vi "WordOfTheDay.vi"() -> ()   [LabVIEW 2018]
uses:
  State.ctl
  <vilib>/Utility/error.llb/Error Cluster From Error Code.vi
  <vilib>/ErrorRing/Error Ring.xnode
  MerriamWebsterJSON.lvlib
panel:
  out "error out":errorcluster
  in  "error in (no error)":errorcluster
  out "Audio Found?":bool
  in  "Play Sound":bool
  in  "Get Word":bool
  out "Output":string
  in  "Stop":bool
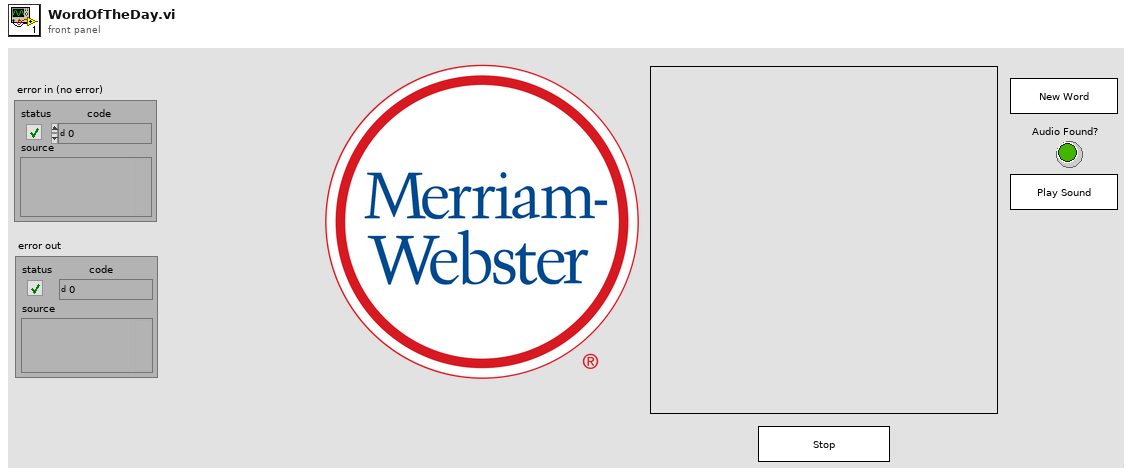
[diagram p1: front panel]
types:
  T1 = typedef "State.ctl" = enum16{"Init", "Wait", "Get Definition", "Get Sound", "Play Sound", "Shutdown"}
  T2 = enum8{"Enabled", "Disabled", "Disabled and Grayed Out"}
  T3 = typedef "LabVIEWHTTPClient.lvlib/ClientHandle.ctl" = refnum<k1>
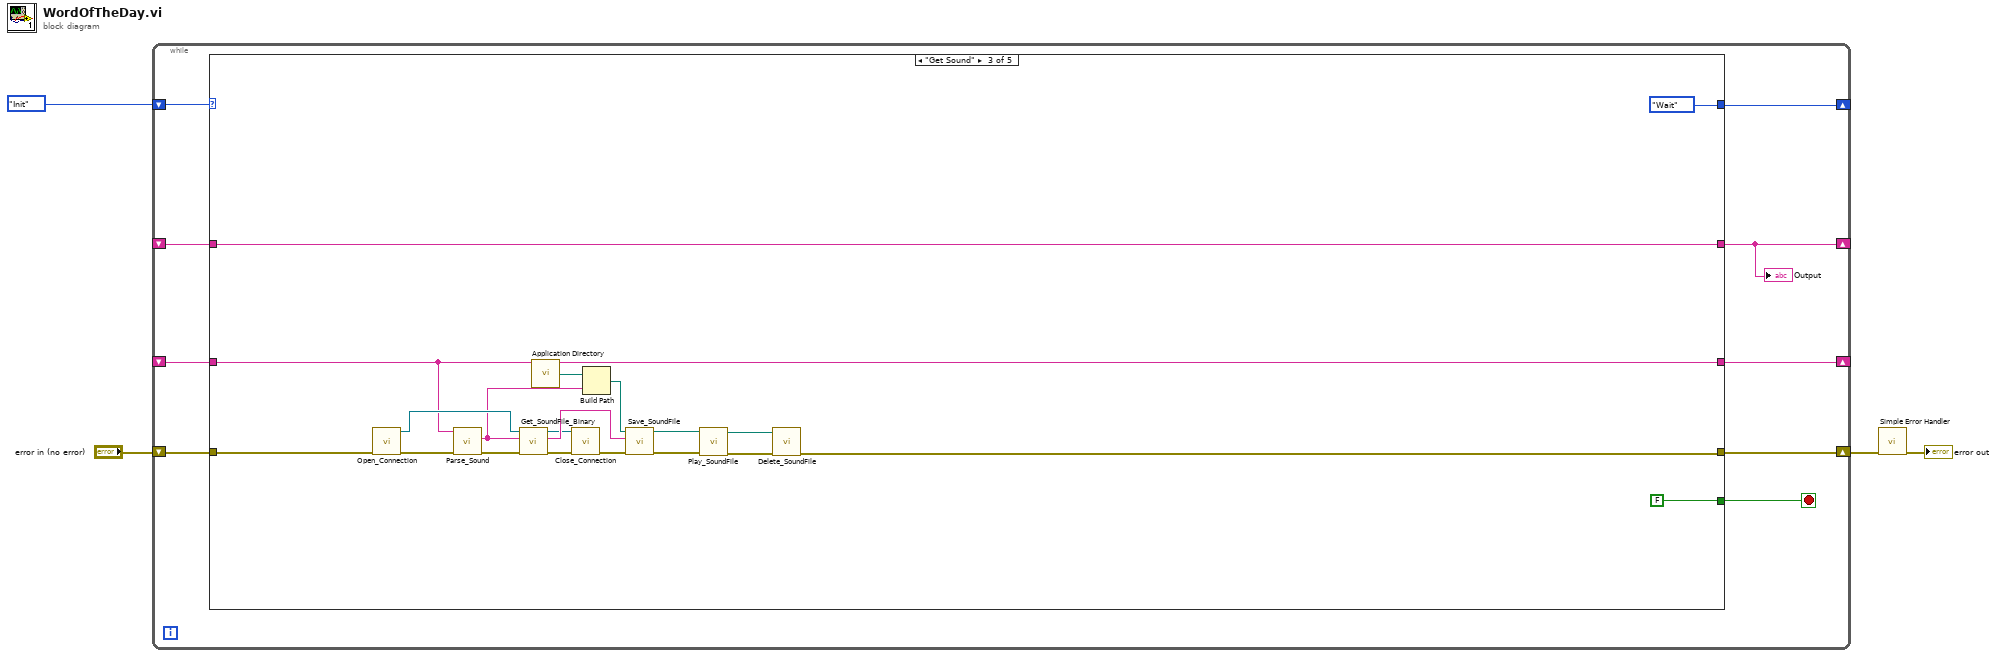
[diagram p0: block diagram]
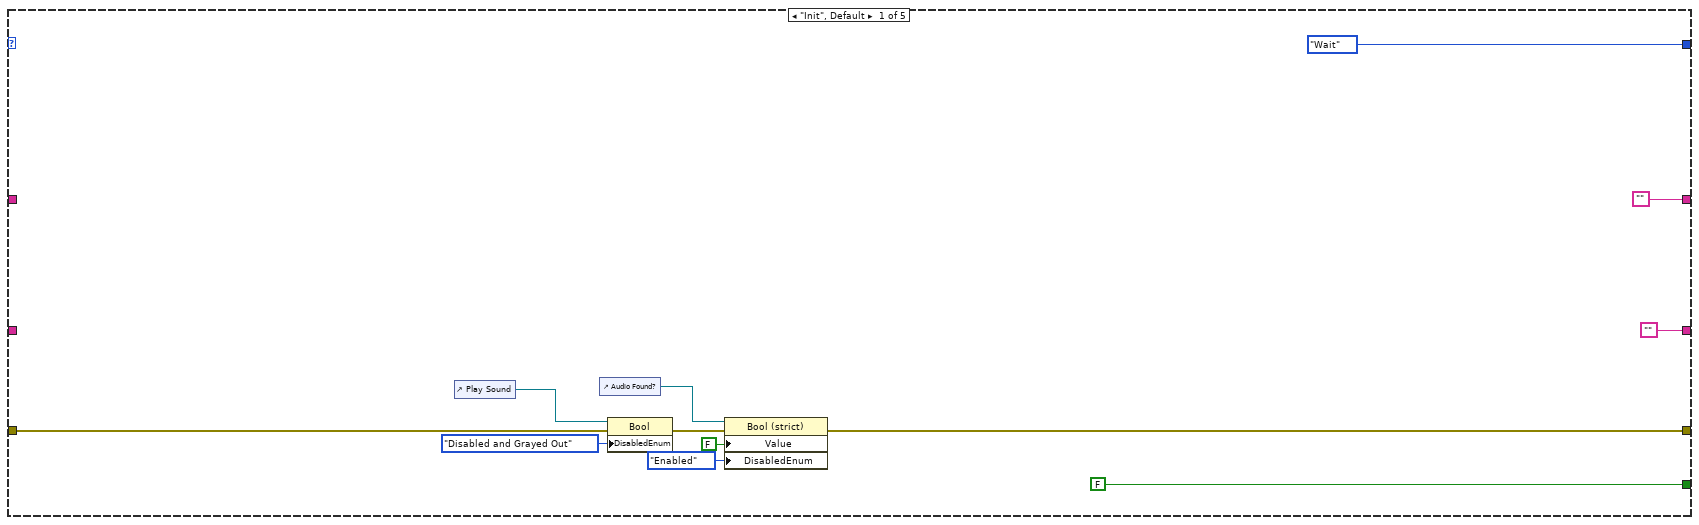
[diagram p2: hidden frame]
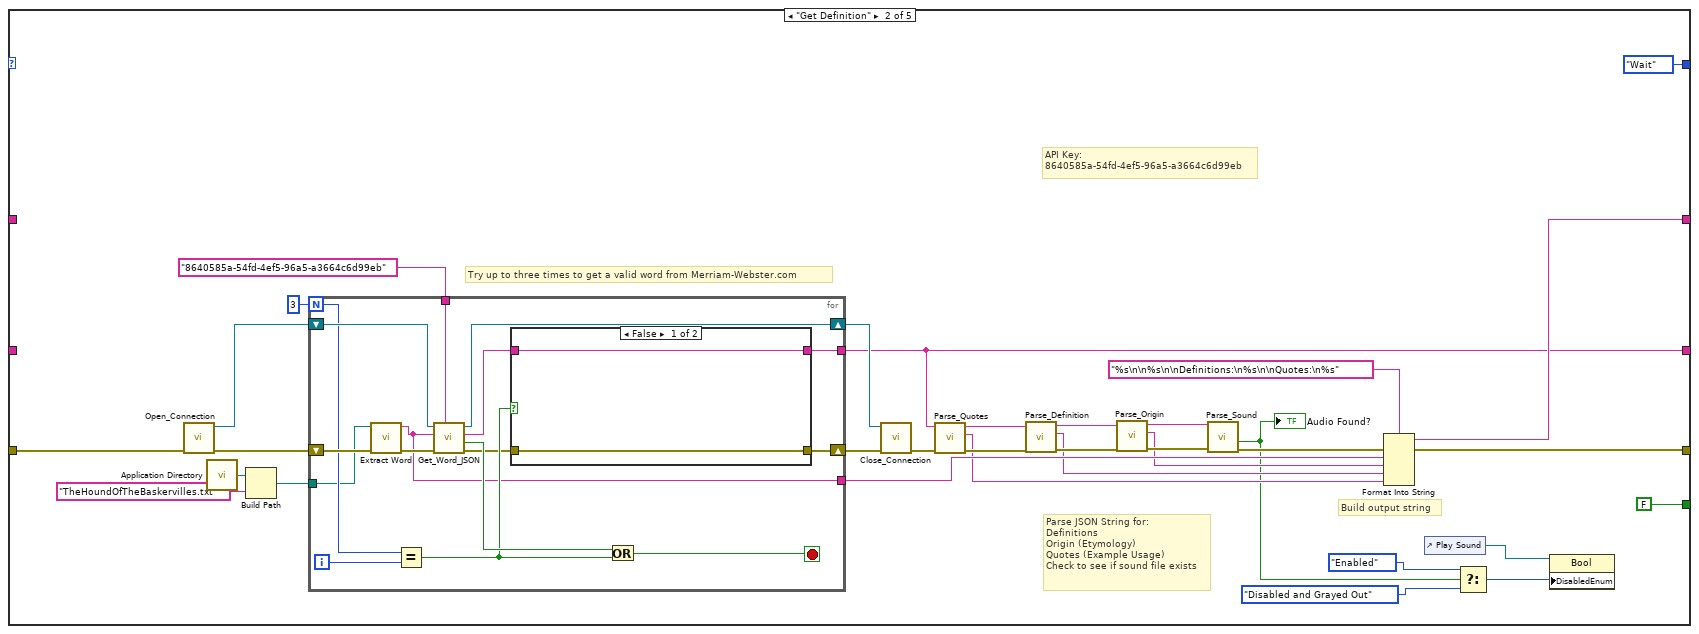
[diagram p3: hidden frame]
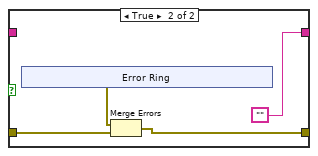
[diagram p4: hidden frame]
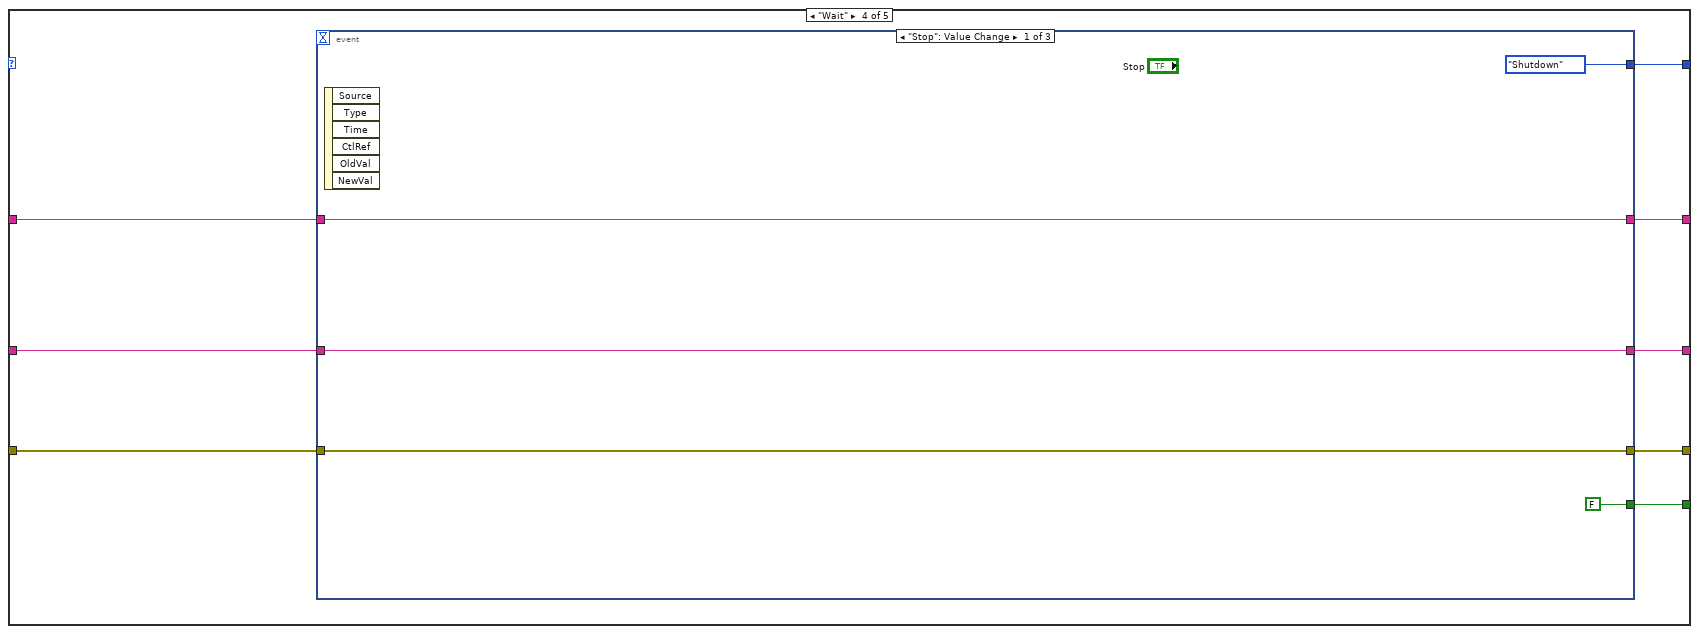
[diagram p5: hidden frame]
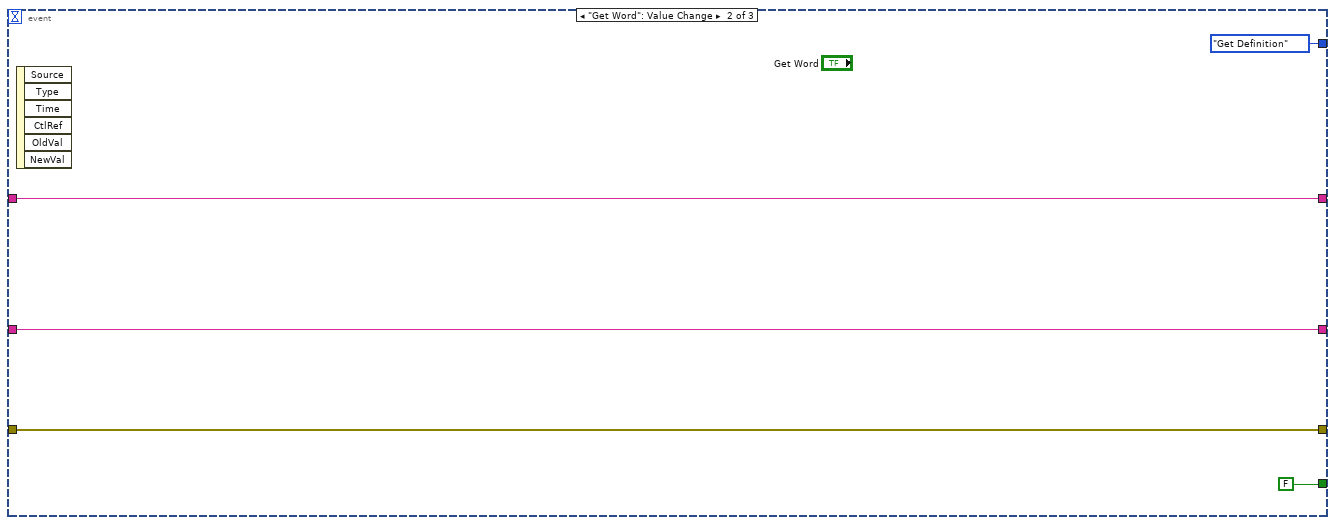
[diagram p6: hidden frame]
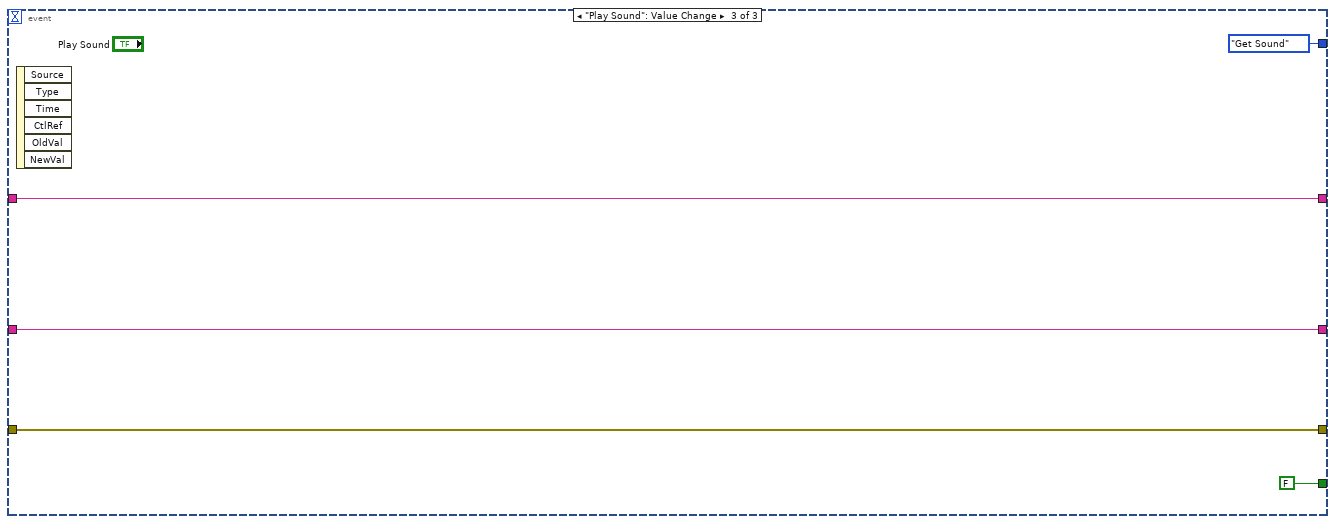
[diagram p7: hidden frame]
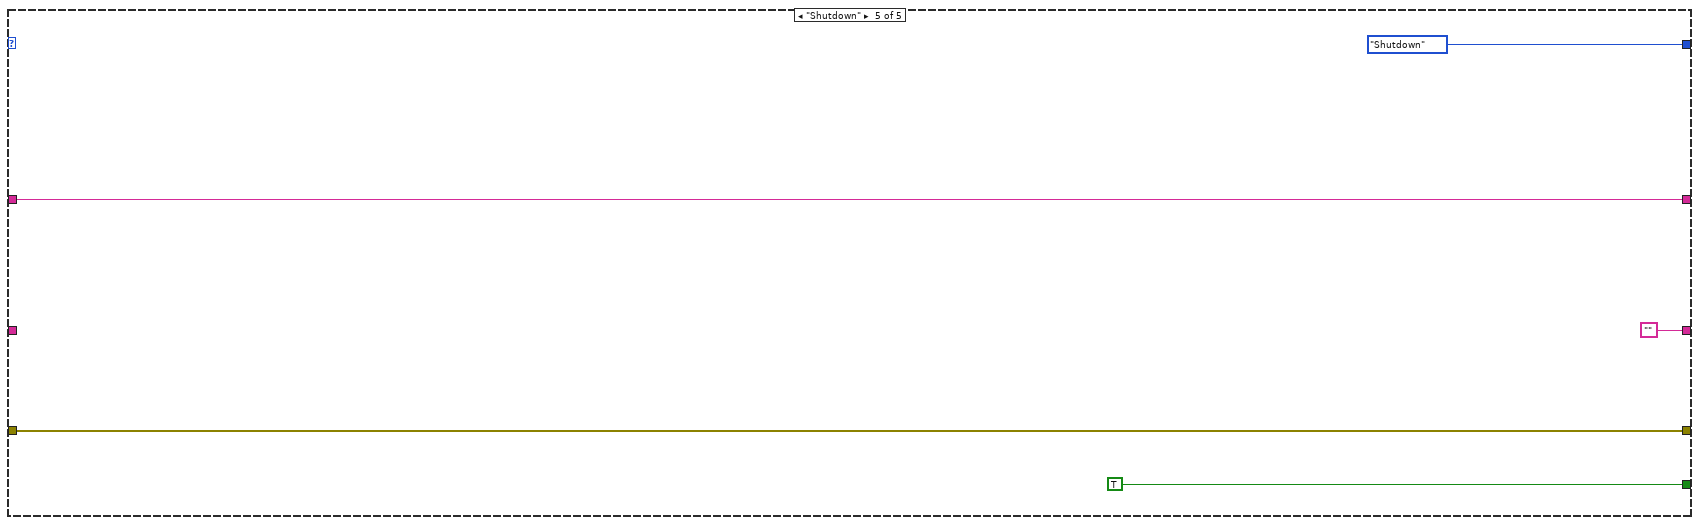
[diagram p8: hidden frame]
diagram:
  n1 = while {
    shift-right: [w12] -> _
    shift-left: State."Init" -> [w13]
    shift-right: [w9] -> _
    shift-left: _ -> [w8]
    shift-right: [w7] -> w2
    shift-left: "error in (no error)" -> [w10]
    shift-right: [w6] -> _
    shift-left: _ -> [w5]
    stop <- w11 stop-if-true
    n2 = case shown="\"Get Sound\"" w13 {
      tunnel: [State."Wait" State."Wait" State."Wait" w112 State."Shutdown"] -> w12
      tunnel: [FALSE FALSE FALSE w113 TRUE] -> w11
      tunnel: w10 -> [w19 w53 w103 w111 w130]
      tunnel: ["" w39 w91 w106 w129] -> w9
      tunnel: w8 -> [_ _ w91 w107 w129]
      tunnel: [w18 w34 w87 w110 w130] -> w7
      tunnel: ["" w35 w90 w108 ""] -> w6
      tunnel: w5 -> [_ _ w90 w109 _]
      frame "Init", Default {
        n3 = control-ref of="Play Sound"() -> (w21:refnum<vi>)
        n4 = control-ref of="Audio Found?"() -> (w17:refnum<vi>)
        n5 = property class="Bool"(reference=w21, error in=w19, "DisabledEnum"=T2."Disabled and Grayed Out" ("Disabled")) -> (error out=w20:errorcluster)  [unwired: 1 out]
        n6 = property class="Bool (strict)"(reference=w17, error in=w20, "Value"=FALSE, "DisabledEnum"=T2."Enabled" ("Disabled")) -> (error out=w18:errorcluster)  [unwired: 1 out]
      }
      frame "Get Definition" {
        # "Build output string"
        # "Parse JSON String for:\nDefinitions\nOrigin (Etymology)\nQuotes (Example Usage)\nCheck to see if sound file exists"
        # "Try up to three times to get a valid word from Merriam-Webster.com"
        # "API Key:\n8640585a-54fd-4ef5-96a5-a3664c6d99eb"
        n7 = call "Open_Connection.vi"("error in (no error)"=w53) -> ("error out"=w55:errorcluster, "client handle out"=w54:T3)  [unwired: 9 in]
        n8 = call <vilib>:"Application Directory.vi"() -> ("Application Directory"=w28:path)
        n9 = Build Path(base path=w28, name or relative path="TheHoundOfTheBaskervilles.txt") -> (appended path=w26:path)
        n10 = for {
          N: 3 -> [w68]
          tunnel: "8640585a-54fd-4ef5-96a5-a3664c6d99eb" -> [w74]
          shift-right: [w61] -> w37
          shift-left: w55 -> [w71]
          shift-right: [w66] -> w38
          shift-left: w54 -> [w73]
          tunnel: [w64] -> w35
          tunnel: [w60] -> w49
          tunnel: w26 -> [w59]
          i -> [w67]
          stop <- w70 stop-if-true
          n11 = call "Extract Word.vi"("error in (no error)"=w71, "file path (use dialog)"=w59) -> ("error out"=w72:errorcluster, "Random Word"=w60:string)  [unwired: 8 in]
          n12 = Equal?(x=w68, y=w67) -> (x = y?=w63:bool)
          n13 = call "Get_Word_JSON.vi"("API Key"=w74, "error in (no error)"=w72, "Word"=w60, "client handle"=w73) -> ("error out"=w62:errorcluster, "Valid Definition?"=w69:bool, "body"=w65:string, "client handle out"=w66:T3)  [unwired: 4 in]
          n14 = case shown="False" w63 {
            tunnel: w65 -> [w76 _]
            tunnel: [w76 ""] -> w64
            tunnel: w62 -> [w75 w80]
            tunnel: [w75 w78] -> w61
            frame False {
            }
            frame True {
              n15 = xnode "Error Ring"() -> ("error out"=w77:errorcluster)
              n16 = Merge Errors(w77, w80) -> (w78:errorcluster)
            }
          }
          n17 = Or(x=w69, y=w63) -> (x .or. y?=w70:bool)
        }
        n18 = call "Close_Connection.vi"("error in (no error)"=w37, "Session In"=w38) -> ("error out"=w36:errorcluster)  [unwired: 9 in]
        n19 = call "Parse_Quotes.vi"("error in (no error)"=w36, "JSON String In"=w35) -> ("error out"=w47:errorcluster, "Examples"=w40:string, "JSON String Out"=w48:string)  [unwired: 6 in, 1 out]
        n20 = call "Parse_Definition.vi"("error in (no error)"=w47, "JSON String In"=w48) -> ("error out"=w45:errorcluster, "Definition(s)"=w41:string, "JSON String Out"=w46:string)  [unwired: 6 in, 1 out]
        n21 = call "Parse_Origin.vi"("error in (no error)"=w45, "JSON String In"=w46) -> ("error out"=w43:errorcluster, "Origin"=w42:string, "JSON String Out"=w44:string)  [unwired: 6 in, 1 out]
        n22 = call "Parse_Sound.vi"("error in (no error)"=w43, "JSON String"=w44) -> ("error out"=w50:errorcluster, "Found?"=w32:bool)  [unwired: 6 in, 2 out]
        "Audio Found?" <- w32
        n23 = Format Into String(format string="%s\n\n%s\n\nDefinitions:\n%s\n\nQuotes:\n%s", error in=w50, w49, w42, w41, w40) -> (resulting string=w39:string, error out=w34:errorcluster)  [unwired: 1 in]
        n24 = control-ref of="Play Sound"() -> (w33:refnum<vi>)
        n25 = Select(t=T2."Enabled" ("Disabled"), s=w32, f=T2."Disabled and Grayed Out" ("Disabled")) -> (s? t:f=w31:T2)
        n26 = property class="Bool"(reference=w33, "DisabledEnum"=w31) -> ()  [unwired: 1 in, 2 out]
      }
      frame "Get Sound" {
        n27 = call "Open_Connection.vi"("error in (no error)"=w103) -> ("error out"=w101:errorcluster, "client handle out"=w102:T3)  [unwired: 9 in]
        n28 = call "Parse_Sound.vi"("error in (no error)"=w101, "JSON String"=w90) -> ("error out"=w100:errorcluster, "Sound File Name"=w86:string)  [unwired: 6 in, 2 out]
        n29 = call "Get_SoundFile_Binary.vi"("error in (no error)"=w100, "Sound File Name"=w86, "Session In"=w102) -> ("error out"=w93:errorcluster, "Binary String"=w99:string, "Session Out"=w94:T3)  [unwired: 6 in]
        n30 = call <vilib>:"Application Directory.vi"() -> ("Application Directory"=w98:path)
        n31 = call "Close_Connection.vi"("error in (no error)"=w93, "Session In"=w94) -> ("error out"=w92:errorcluster)  [unwired: 9 in]
        n32 = Build Path(base path=w98, name or relative path=w86) -> (appended path=w97:path)
        n33 = call "Save_SoundFile.vi"("error in"=w92, "Binary String"=w99, "File Path In"=w97) -> ("error out"=w95:errorcluster, "File Path Out"=w96:path)  [unwired: 7 in]
        n34 = call "Play_SoundFile.vi"("error in (no error)"=w95, "File Path In"=w96) -> ("error out"=w88:errorcluster, "File Path Out"=w89:path)  [unwired: 8 in]
        n35 = call "Delete_SoundFile.vi"("error in (no error)"=w88, "File Path In"=w89) -> ("error out"=w87:errorcluster)  [unwired: 9 in]
      }
      frame "Wait" {
        n36 = event shown="[0] \"Stop\": Value Change" {
          selector: _ -> [_ _ _]
          dyn-events: _ -> [_ _ _]
          timeout: _ -> [_ _ _]
          tunnel: [FALSE FALSE FALSE] -> w113
          tunnel: [State."Shutdown" State."Get Definition" State."Get Sound"] -> w112
          tunnel: w111 -> [w114 w122 w124]
          tunnel: [w114 w122 w124] -> w110
          tunnel: w109 -> [w115 w121 w125]
          tunnel: [w115 w121 w125] -> w108
          tunnel: w107 -> [w116 w120 w126]
          tunnel: [w116 w120 w126] -> w106
          event "Stop": Value Change {
            n37 = event-data() -> ()  [unwired: 1 in, 6 out]
          }
          event "Get Word": Value Change {
            n38 = event-data() -> ()  [unwired: 1 in, 6 out]
          }
          event "Play Sound": Value Change {
            n39 = event-data() -> ()  [unwired: 1 in, 6 out]
          }
        }
      }
      frame "Shutdown" {
      }
    }
    "Output" <- w9
  }
  n40 = call <vilib>:"Simple Error Handler.vi"("error in (no error)"=w2) -> ("error out"=→"error out":errorcluster)  [unwired: 4 in, 4 out]
